vi "Planner_Creator.vi"(8 "error in (no error)":errorcluster) -> (0 "error out":errorcluster)   [LabVIEW 2017]
uses:
  <vilib>/Utility/file.llb/Read Delimited Spreadsheet (string).vi
  <vilib>/Utility/file.llb/Write Delimited Spreadsheet (string).vi
panel:
  out "Table":string[][](table)
  in  "BLOCK No":string(combo)
  in  "Delete Button":bool
  in  "Save Button":bool
  in  "Qty":u16=1 min=1 max=90 step=1
  in  "HOME":bool
  in  "UPDATE TABLE":bool
  in  "FG CAT No":string(combo)
  # "Plan Creater"
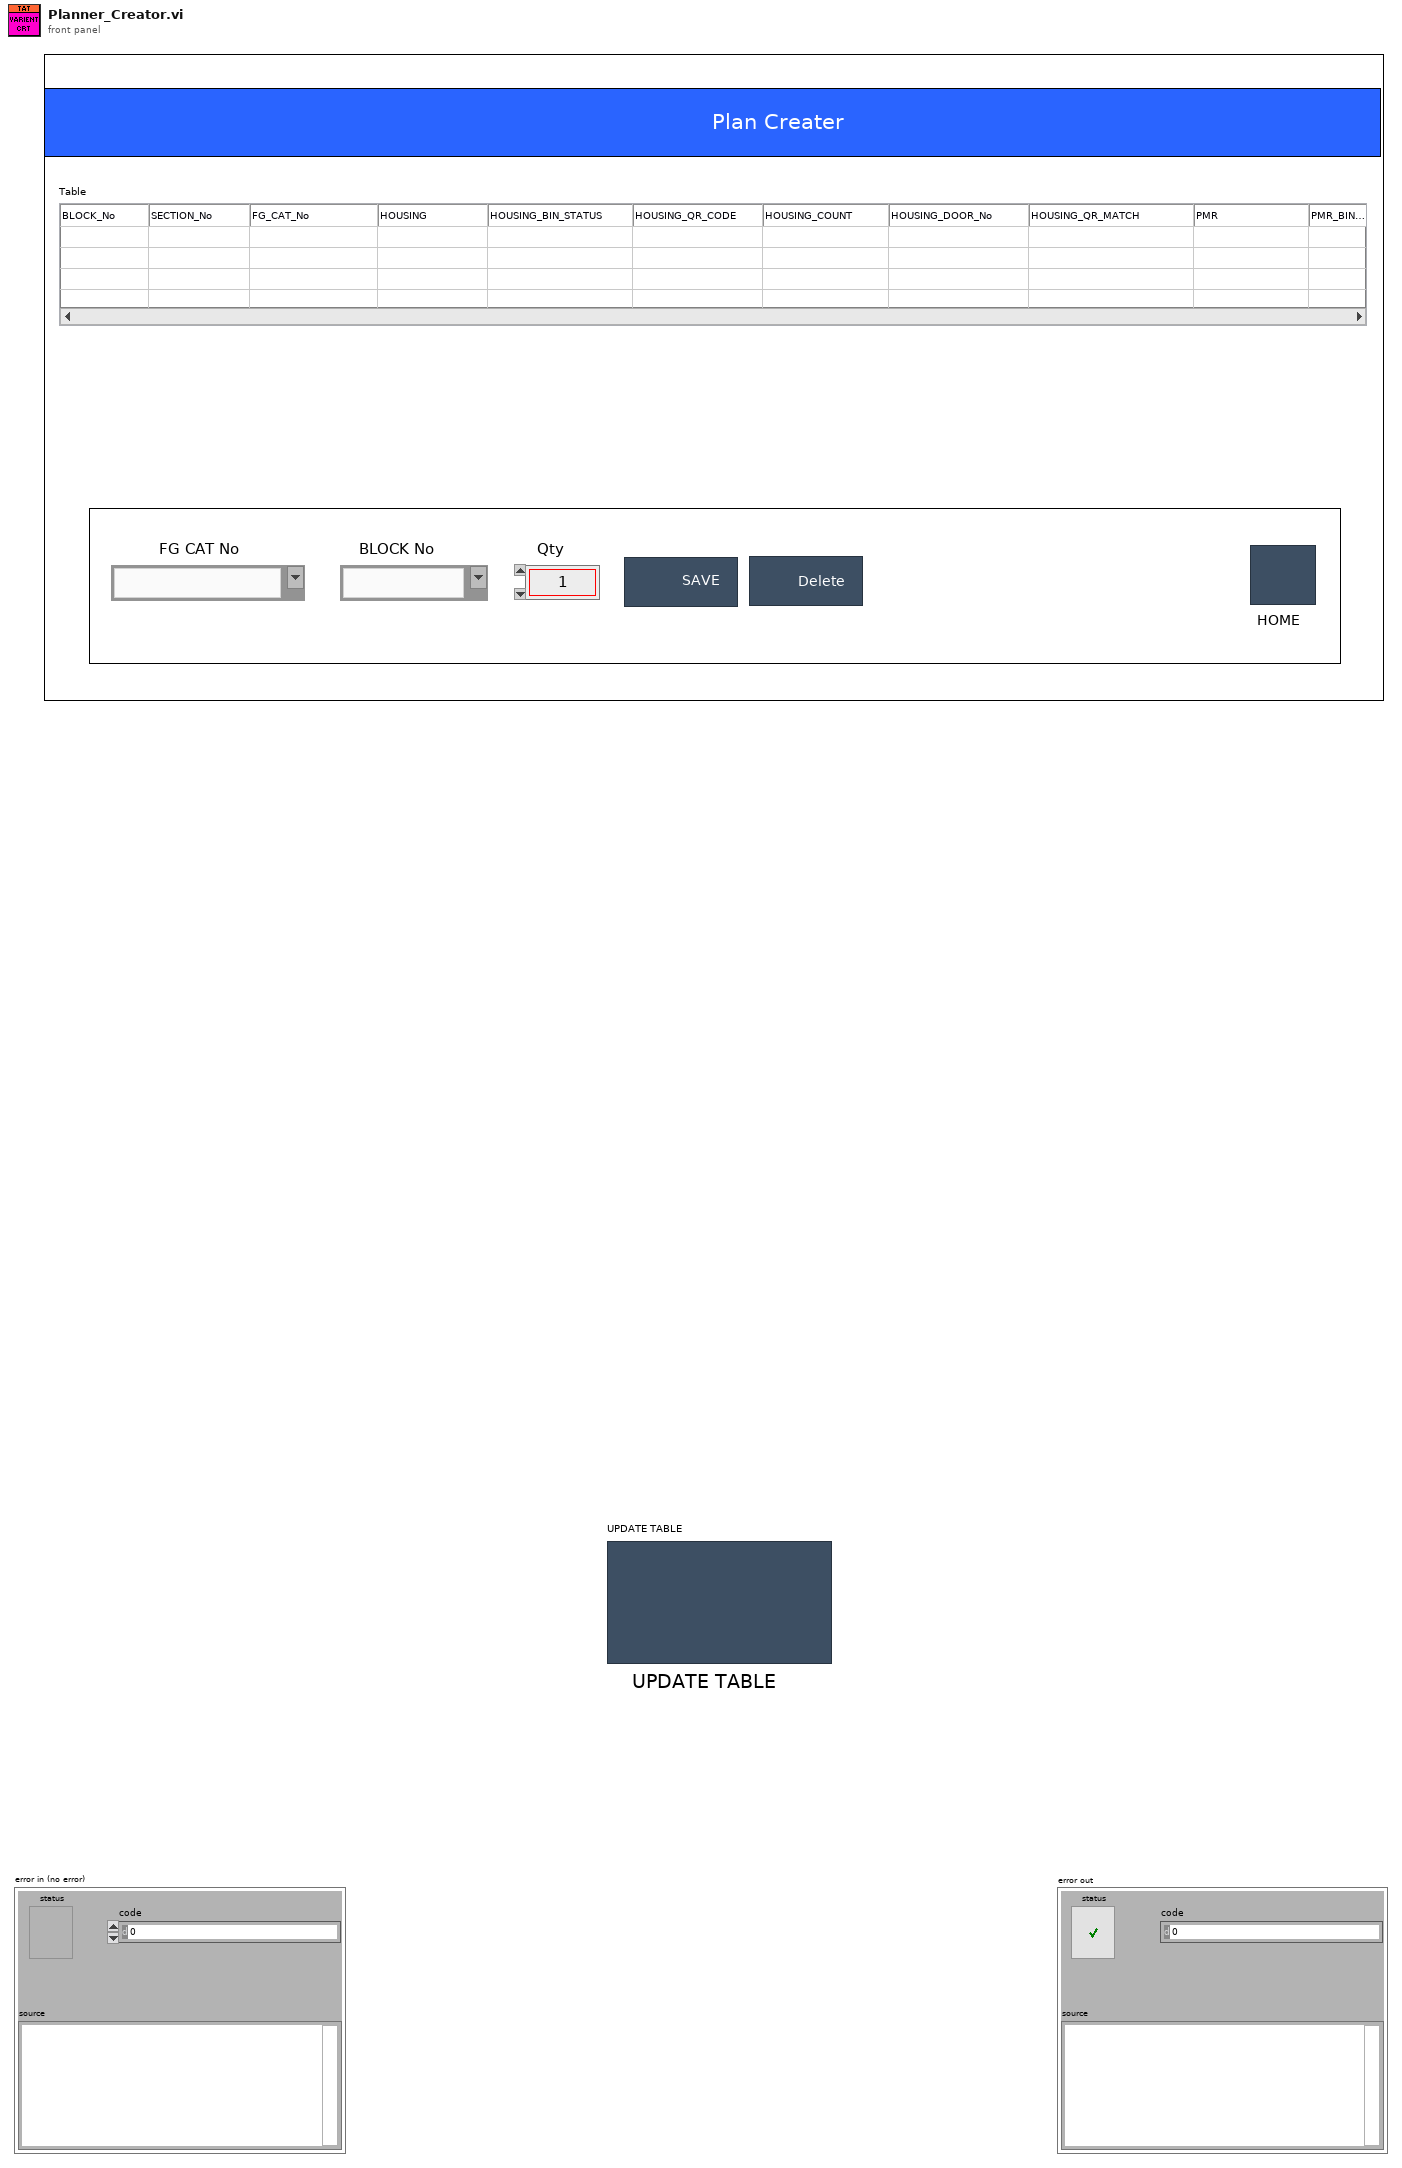
[diagram p1: front panel]
types:
  T1 = enum32{"invalid app kind", "Development System", "Run Time System", "Student Edition", "Embedded LabVIEW", "Evaluation", "Custom"}
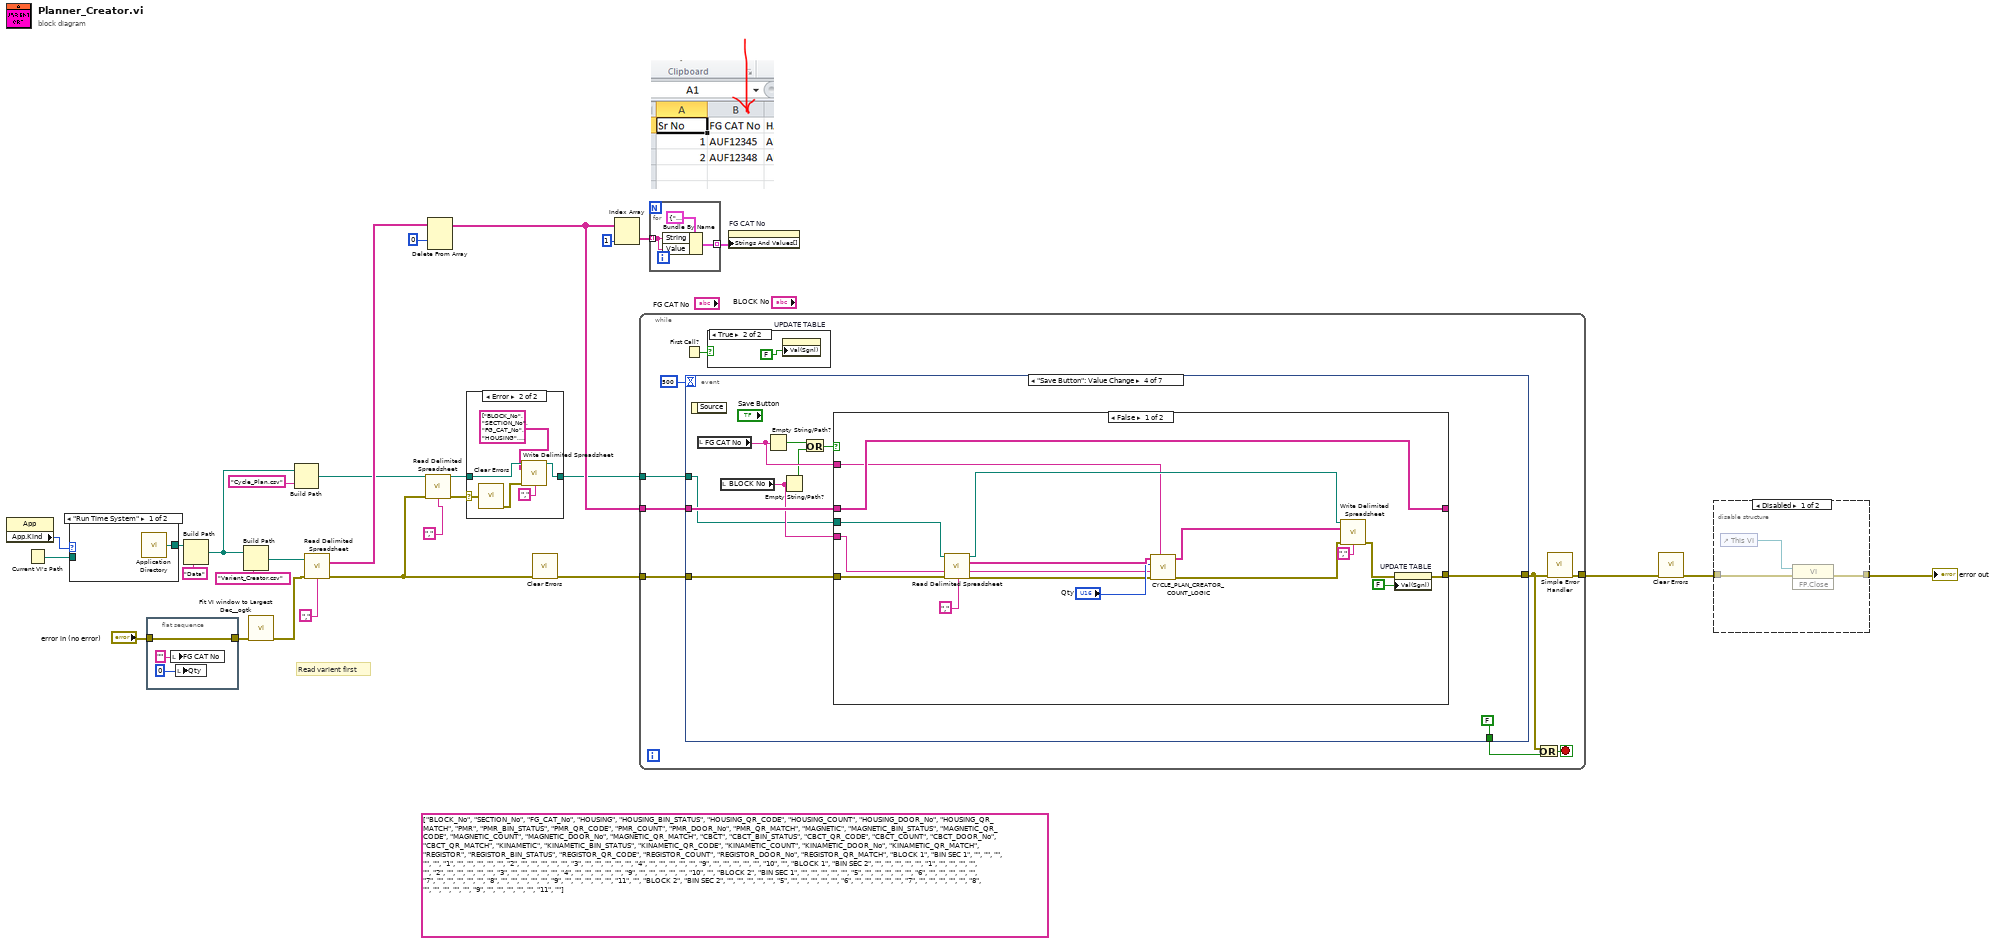
[diagram p0: block diagram]
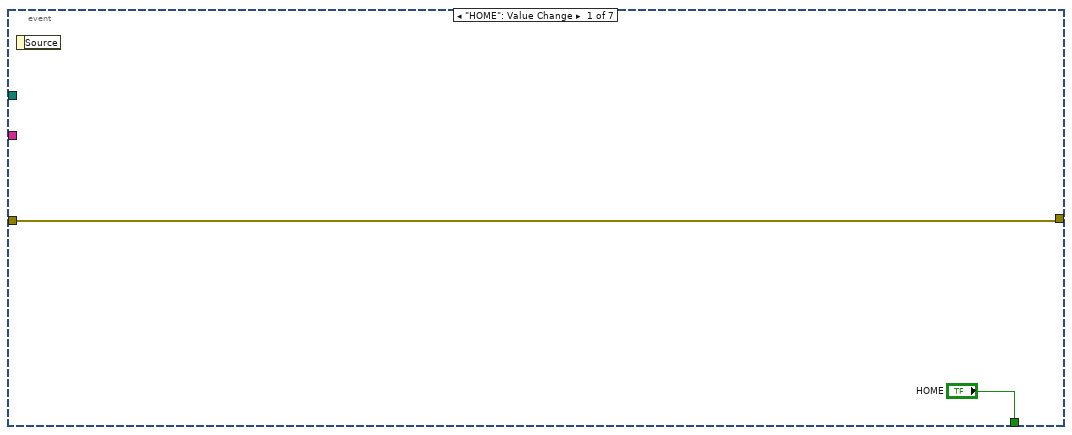
[diagram p4: hidden frame]
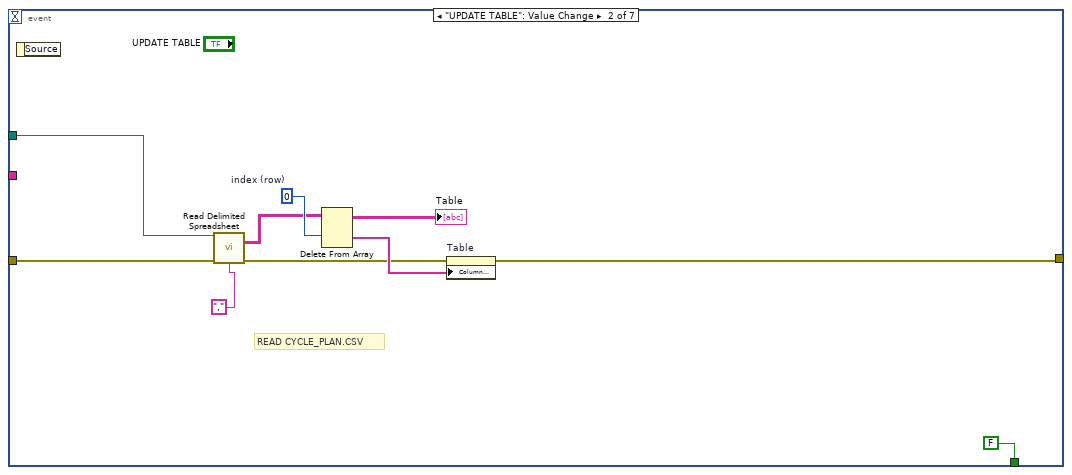
[diagram p5: hidden frame]
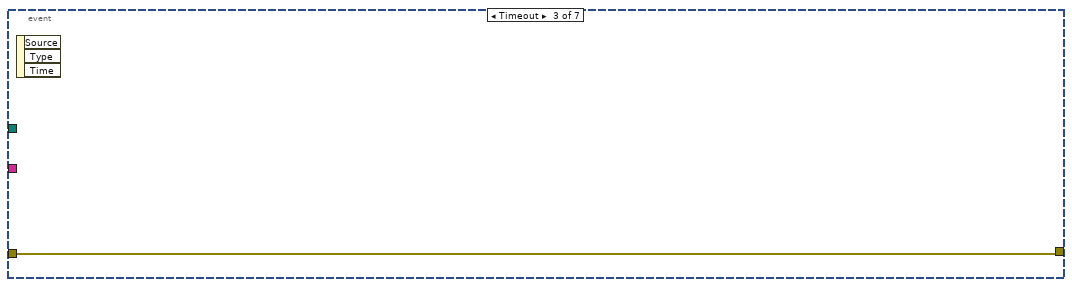
[diagram p6: hidden frame]
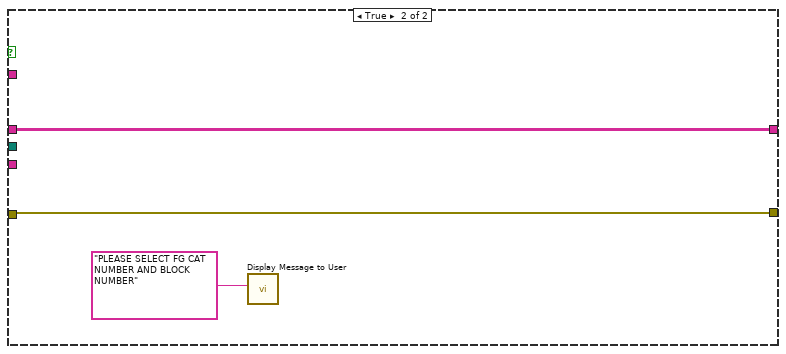
[diagram p7: hidden frame]
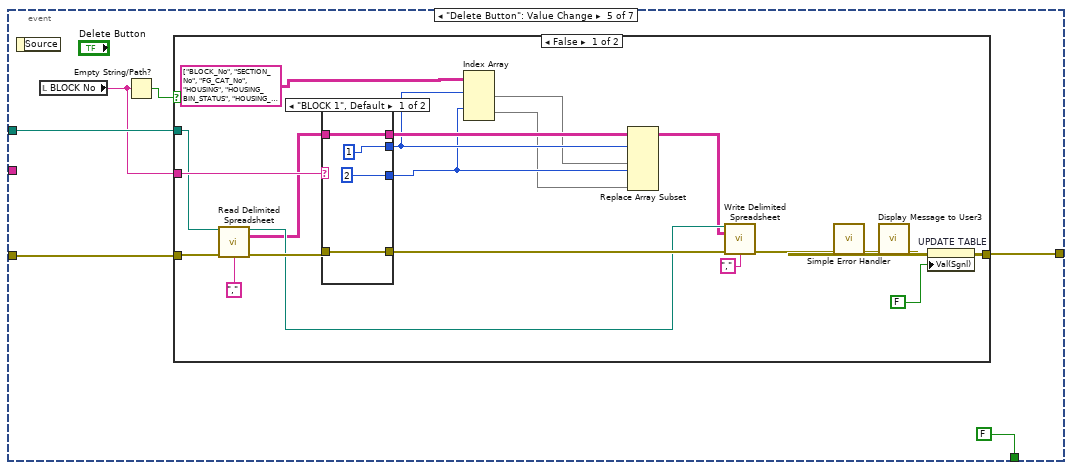
[diagram p8: hidden frame]
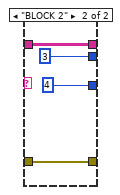
[diagram p9: hidden frame]
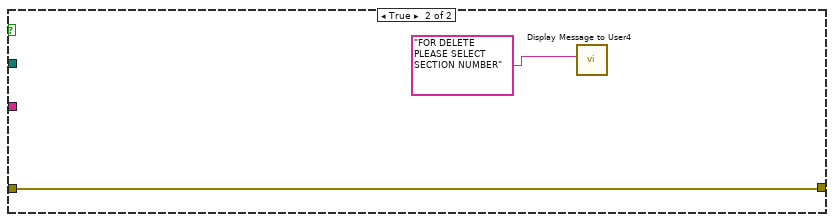
[diagram p10: hidden frame]
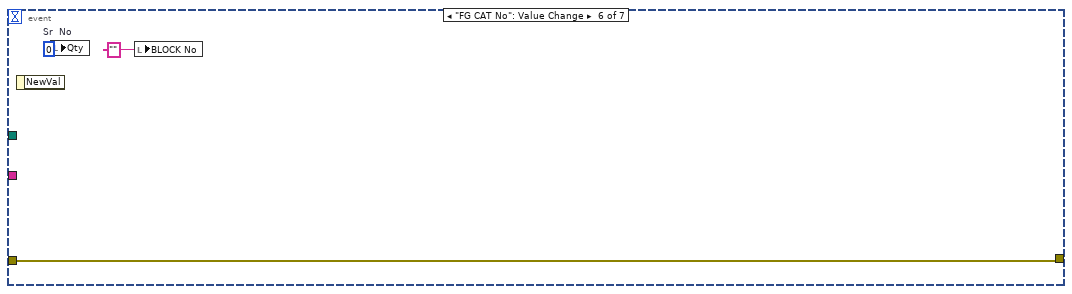
[diagram p11: hidden frame]
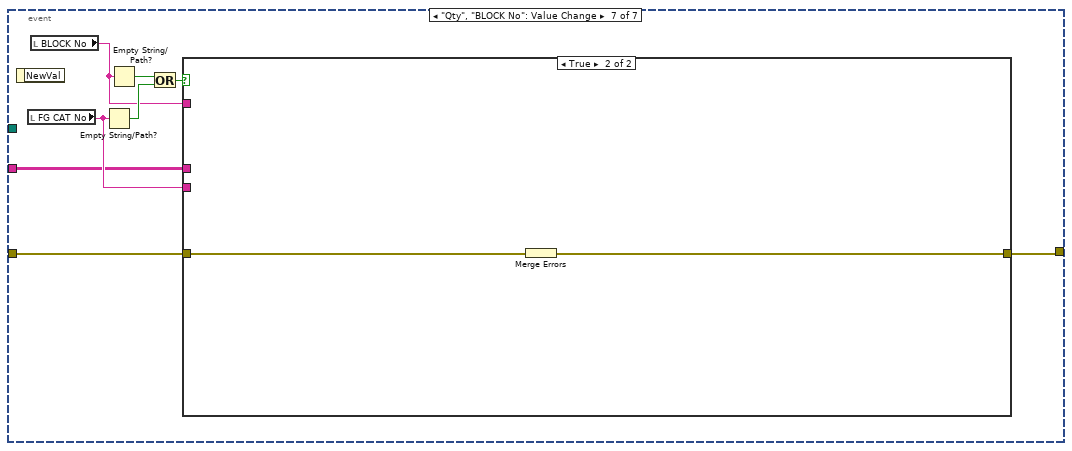
[diagram p12: hidden frame]
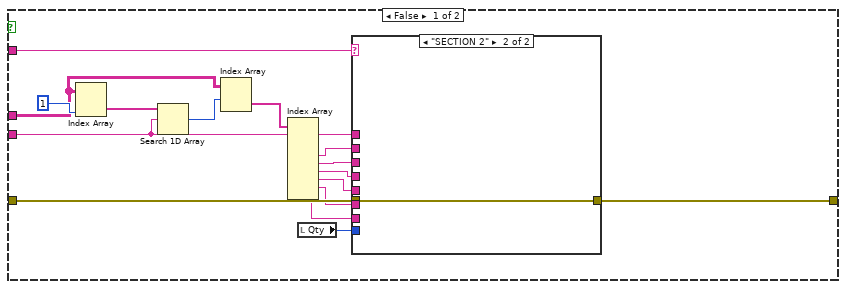
[diagram p13: hidden frame]
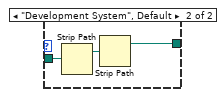
[diagram p16: hidden frame]
diagram:
  (unwired) string[][] [["BLOCK_No", "SECTION_No", "FG_CAT_No", "HOUSING", "HOUSING_BIN_STATUS", "HOUSING_QR_CODE", "HOUSING_COUNT", "HOUSING_DOOR_No", "HOUSING_QR_MATCH", "PMR", "PMR_BIN_STATUS", "PMR_QR_CODE", "PMR_COUNT", "PMR_DOOR_No", "PMR_QR_MATCH", "MAGNETIC", "MAGNETIC_BIN_STATUS", "MAGNETIC_QR_CODE", "MAGNETIC_COUNT", "MAGNETIC_DOOR_No", "MAGNETIC_QR_MATCH", "CBCT", "CBCT_BIN_STATUS", "CBCT_QR_CODE", "CBCT_COUNT", "CBCT_DOOR_No", "CBCT_QR_MATCH", "KINAMETIC", "KINAMETIC_BIN_STATUS", "KINAMETIC_QR_CODE", "KINAMETIC_COUNT", "KINAMETIC_DOOR_No", "KINAMETIC_QR_MATCH", "REGISTOR", "REGISTOR_BIN_STATUS", "REGISTOR_QR_CODE", "REGISTOR_COUNT", "REGISTOR_DOOR_No", "REGISTOR_QR_MATCH"], ["BLOCK 1", "BIN SEC 1", "", "", "", "", "", "1", "", "", "", "", "", "2", "", "", "", "", "", "3", "", "", "", "", "", "4", "", "", "", "", "", "9", "", "", "", "", "", "10", ""], ["BLOCK 1", "BIN SEC 2", "", "", "", "", "", "1", "", "", "", "", "", "2", "", "", "", "", "", "3", "", "", "", "", "", "4", "", "", "", "", "", "9", "", "", "", "", "", "10", ""], ["BLOCK 2", "BIN SEC 1", "", "", "", "", "", "5", "", "", "", "", "", "6", "", "", "", "", "", "7", "", "", "", "", "", "8", "", "", "", "", "", "9", "", "", "", "", "", "11", ""], ["BLOCK 2", "BIN SEC 2", "", "", "", "", "", "5", "", "", "", "", "", "6", "", "", "", "", "", "7", "", "", "", "", "", "8", "", "", "", "", "", "9", "", "", "", "", "", "11", ""]]
  # "Read varient first"
  n1 = property class="App"() -> ("App.Kind"=w22:T1)  [unwired: 2 in, 2 out]
  n2 = Current VI's Path() -> (path=w23:path)
  n3 = case shown="\"Run Time System\"" w22 {
    tunnel: w23 -> [_ w31]
    tunnel: [w29 w30] -> w19
    frame "Run Time System" {
      n4 = call <vilib>:"Application Directory.vi"() -> ("Application Directory"=w29:path)
    }
    frame "Development System", Default {
      n5 = Strip Path(path=w31) -> (stripped path=w32:path)  [unwired: 1 out]
      n6 = Strip Path(path=w32) -> (stripped path=w30:path)  [unwired: 1 out]
    }
  }
  n7 = flat-sequence {
    tunnel: [w35] -> w24
    tunnel: "error in (no error)" -> [w35]
    frame #0 {
      n8 = local write "FG CAT No"("" ("PART NUMBER")) -> ()
      n9 = local write "Qty"(u16 0 ("BATCH SIZE")) -> ()
    }
  }
  n10 = Build Path(base path=w19, name or relative path="Data") -> (appended path=w20:path)
  n11 = Build Path(base path=w20, name or relative path="Varient_Creator.csv") -> (appended path=w2:path)
  n12 = call <userlib>:"Fit VI window to Largest Dec__ogtk.vi"("error in (no error)"=w24) -> ("error out"=w18:errorcluster)  [unwired: 5 in, 1 out]
  n13 = Build Path(base path=w20, name or relative path="Cycle_Plan.csv") -> (appended path=w8:path)
  n14 = call-poly <vilib>:"Read Delimited Spreadsheet.vi"("file path (dialog if empty)"=w2, "error in (no error)"=w18, "delimiter (\\t)"=",") -> ("all rows"=w16:string[][], "error out"=w9:errorcluster)  [unwired: 7 in, 4 out]
  n15 = call-poly <vilib>:"Read Delimited Spreadsheet.vi"("file path (dialog if empty)"=w8, "error in (no error)"=w9, "delimiter (\\t)"=",") -> ("new file path (Not A Path if cancelled)"=w4:path, "error out"=w6:errorcluster)  [unwired: 7 in, 4 out]
  n16 = Delete From Array(array=w16, index (row)=0) -> (array with subset deleted=w11:string[][])  [unwired: 2 in, 1 out]
  n17 = case shown="Error" w6 {
    selector: w6 -> [_ w39]
    tunnel: [w36 w40] -> w5
    tunnel: w4 -> [w36 w41]
    frame No Error {
    }
    frame Error {
      n18 = call <vilib>:"Clear Errors.vi"("error in (no error)"=w39) -> ("error out"=w38:errorcluster)  [unwired: 5 in, 1 out]
      n19 = call-poly <vilib>:"Write Delimited Spreadsheet.vi"("file path (dialog if empty)"=w41, "2D data"=string[][] [["BLOCK_No", "SECTION_No", "FG_CAT_No", "HOUSING", "HOUSING_BIN_STATUS", "HOUSING_QR_CODE", "HOUSING_COUNT", "HOUSING_DOOR_No", "HOUSING_QR_MATCH", "PMR", "PMR_BIN_STATUS", "PMR_QR_CODE", "PMR_COUNT", "PMR_DOOR_No", "PMR_QR_MATCH", "MAGNETIC", "MAGNETIC_BIN_STATUS", "MAGNETIC_QR_CODE", "MAGNETIC_COUNT", "MAGNETIC_DOOR_No", "MAGNETIC_QR_MATCH", "CBCT", "CBCT_BIN_STATUS", "CBCT_QR_CODE", "CBCT_COUNT", "CBCT_DOOR_No", "CBCT_QR_MATCH", "KINAMETIC", "KINAMETIC_BIN_STATUS", "KINAMETIC_QR_CODE", "KINAMETIC_COUNT", "KINAMETIC_DOOR_No", "KINAMETIC_QR_MATCH", "REGISTOR", "REGISTOR_BIN_STATUS", "REGISTOR_QR_CODE", "REGISTOR_COUNT", "REGISTOR_DOOR_No", "REGISTOR_QR_MATCH"], ["BLOCK 1", "BIN SEC 1", "", "", "", "", "", "1", "", "", "", "", "", "2", "", "", "", "", "", "3", "", "", "", "", "", "4", "", "", "", "", "", "9", "", "", "", "", "", "10", ""], ["BLOCK 1", "BIN SEC 2", "", "", "", "", "", "1", "", "", "", "", "", "2", "", "", "", "", "", "3", "", "", "", "", "", "4", "", "", "", "", "", "9", "", "", "", "", "", "10", ""], ["BLOCK 2", "BIN SEC 1", "", "", "", "", "", "5", "", "", "", "", "", "6", "", "", "", "", "", "7", "", "", "", "", "", "8", "", "", "", "", "", "9", "", "", "", "", "", "11", ""], ["BLOCK 2", "BIN SEC 2", "", "", "", "", "", "5", "", "", "", "", "", "6", "", "", "", "", "", "7", "", "", "", "", "", "8", "", "", "", "", "", "9", "", "", "", "", "", "11", ""]], "error in (no error)"=w38, "delimiter (\\t)"=",") -> ("new file path (Not A Path if cancelled)"=w40:path)  [unwired: 10 in, 1 out]
    }
  }
  n20 = call <vilib>:"Clear Errors.vi"("error in (no error)"=w9) -> ("error out"=w10:errorcluster)  [unwired: 5 in, 1 out]
  n21 = Index Array(array=w11, index (col)=1) -> (element=w13:string[])  [unwired: 1 in]
  n22 = while {
    tunnel: [w46] -> w26
    tunnel: w10 -> [w48]
    tunnel: w11 -> [w44]
    tunnel: w5 -> [w43]
    stop <- w50 stop-if-true
    n23 = First Call?() -> (First Call?: T/F=w49:bool)
    n24 = event shown="[3] \"Save Button\": Value Change" {
      selector: _ -> [_ _ _ _ _ _ _]
      dyn-events: _ -> [_ _ _ _ _ _ _]
      timeout: 500 -> [_ _ _ _ _ _ _]
      tunnel: ["HOME" FALSE ("stop") _ FALSE ("stop") FALSE ("stop") _ _] -> w51
      tunnel: [w52 w54 w64 w72 w98 w132 w140] -> w47
      tunnel: w48 -> [w52 w61 w64 w71 w97 w132 w141]
      tunnel: w44 -> [_ _ _ w70 _ _ w134]
      tunnel: w43 -> [_ w60 _ w65 w96 _ _]
      event "HOME": Value Change {
        n25 = event-data() -> ()  [unwired: 1 in, 1 out]
      }
      event "UPDATE TABLE": Value Change {
        w59 = 0  # index (row)
        # "READ CYCLE_PLAN.CSV"
        n26 = event-data() -> ()  [unwired: 1 in, 1 out]
        n27 = call-poly <vilib>:"Read Delimited Spreadsheet.vi"("file path (dialog if empty)"=w60, "error in (no error)"=w61, "delimiter (\\t)"=",") -> ("all rows"=w57:string[][], "error out"=w55:errorcluster)  [unwired: 7 in, 4 out]
        n28 = Delete From Array(array=w57, index (row)=w59) -> (deleted portion=w58:string[], array with subset deleted=→"Table":string[][])  [unwired: 2 in]
        n29 = property on="Table" class="Tbl (strict)"(error in=w55, "Column Headers[]"=w58) -> (error out=w54:errorcluster)  [unwired: 1 in, 1 out]
      }
      event Timeout {
        n30 = event-data() -> ()  [unwired: 1 in, 3 out]
      }
      event "Save Button": Value Change {
        n31 = event-data() -> ()  [unwired: 1 in, 1 out]
        n32 = local read "FG CAT No"() -> (w73:string)
        n33 = local read "BLOCK No"() -> (w66:string)
        n34 = Empty String/Path?(string/path=w73) -> (empty?=w68:bool)
        n35 = Empty String/Path?(string/path=w66) -> (empty?=w69:bool)
        n36 = Or(x=w68, y=w69) -> (x .or. y?=w67:bool)
        n37 = case shown="False" w67 {
          tunnel: [w89 w92] -> w72
          tunnel: w73 -> [w79 _]
          tunnel: w71 -> [w84 w92]
          tunnel: w70 -> [w88 w91]
          tunnel: [w88 w91] -> _
          tunnel: w66 -> [w77 _]
          tunnel: w65 -> [w83 _]
          frame False {
            n38 = call-poly <vilib>:"Read Delimited Spreadsheet.vi"("file path (dialog if empty)"=w83, "error in (no error)"=w84, "delimiter (\\t)"=",") -> ("new file path (Not A Path if cancelled)"=w82:path, "all rows"=w81:string[][], "error out"=w78:errorcluster)  [unwired: 7 in, 3 out]
            n39 = call "CYCLE_PLAN_CREATOR_COUNT_LOGIC.vi"("FG CAT No"=w79, "error in (no error)"=w78, "BLOCK NO"=w77, "Qty"="Qty", "all rows IN"=w81) -> ("error out"=w75:errorcluster, "all rows OUT"=w76:string[][])  [unwired: 5 in]
            n40 = call-poly <vilib>:"Write Delimited Spreadsheet.vi"("file path (dialog if empty)"=w82, "2D data"=w76, "error in (no error)"=w75, "delimiter (\\t)"=",") -> ("error out"=w87:errorcluster)  [unwired: 10 in, 1 out]
            n41 = property on="UPDATE TABLE" class="Bool (strict)"(error in=w87, "Val(Sgnl)"=FALSE) -> (error out=w89:errorcluster)  [unwired: 1 in, 1 out]
          }
          frame True {
            n42 = call "Display Message to User"("Message"="PLEASE SELECT FG CAT NUMBER AND BLOCK NUMBER") -> ()  [unwired: 9 in, 2 out]
          }
        }
      }
      event "Delete Button": Value Change {
        n43 = event-data() -> ()  [unwired: 1 in, 1 out]
        n44 = local read "BLOCK No"() -> (w95:string)
        n45 = Empty String/Path?(string/path=w95) -> (empty?=w94:bool)
        n46 = case shown="False" w94 {
          tunnel: [w119 w129] -> w98
          tunnel: w97 -> [w115 w129]
          tunnel: w95 -> [w116 _]
          tunnel: w96 -> [w112 _]
          frame False {
            n47 = call-poly <vilib>:"Read Delimited Spreadsheet.vi"("file path (dialog if empty)"=w112, "error in (no error)"=w115, "delimiter (\\t)"=",") -> ("new file path (Not A Path if cancelled)"=w108:path, "all rows"=w106:string[][], "error out"=w114:errorcluster)  [unwired: 7 in, 3 out]
            n48 = case shown="\"BLOCK 1\", Default" w116 {
              tunnel: w114 -> [w124 w128]
              tunnel: [w124 w128] -> w110
              tunnel: [w123 w127] -> w107
              tunnel: w106 -> [w123 w127]
              tunnel: [1 ("disabled index (col)") 3 ("disabled index (col)")] -> w104
              tunnel: [2 ("disabled index (col)") 4 ("disabled index (col)")] -> w103
              frame "BLOCK 1", Default {
              }
              frame "BLOCK 2" {
              }
            }
            n49 = Index Array(array=string[][] [["BLOCK_No", "SECTION_No", "FG_CAT_No", "HOUSING", "HOUSING_BIN_STATUS", "HOUSING_QR_CODE", "HOUSING_COUNT", "HOUSING_DOOR_No", "HOUSING_QR_MATCH", "PMR", "PMR_BIN_STATUS", "PMR_QR_CODE", "PMR_COUNT", "PMR_DOOR_No", "PMR_QR_MATCH", "MAGNETIC", "MAGNETIC_BIN_STATUS", "MAGNETIC_QR_CODE", "MAGNETIC_COUNT", "MAGNETIC_DOOR_No", "MAGNETIC_QR_MATCH", "CBCT", "CBCT_BIN_STATUS", "CBCT_QR_CODE", "CBCT_COUNT", "CBCT_DOOR_No", "CBCT_QR_MATCH", "KINAMETIC", "KINAMETIC_BIN_STATUS", "KINAMETIC_QR_CODE", "KINAMETIC_COUNT", "KINAMETIC_DOOR_No", "KINAMETIC_QR_MATCH", "REGISTOR", "REGISTOR_BIN_STATUS", "REGISTOR_QR_CODE", "REGISTOR_COUNT", "REGISTOR_DOOR_No", "REGISTOR_QR_MATCH"], ["BLOCK 1", "BIN SEC 1", "", "", "", "", "", "1", "", "", "", "", "", "2", "", "", "", "", "", "3", "", "", "", "", "", "4", "", "", "", "", "", "9", "", "", "", "", "", "10", ""], ["BLOCK 1", "BIN SEC 2", "", "", "", "", "", "1", "", "", "", "", "", "2", "", "", "", "", "", "3", "", "", "", "", "", "4", "", "", "", "", "", "9", "", "", "", "", "", "10", ""], ["BLOCK 2", "BIN SEC 1", "", "", "", "", "", "5", "", "", "", "", "", "6", "", "", "", "", "", "7", "", "", "", "", "", "8", "", "", "", "", "", "9", "", "", "", "", "", "11", ""], ["BLOCK 2", "BIN SEC 2", "", "", "", "", "", "5", "", "", "", "", "", "6", "", "", "", "", "", "7", "", "", "", "", "", "8", "", "", "", "", "", "9", "", "", "", "", "", "11", ""]], index (row) #1=w104, index (row) #2=w103) -> (element #1=w102:string[], element #2=w101:string[])  [unwired: 2 in]
            n50 = Replace Array Subset(array=w107, new element #1=w102, index (row) #1=w104, new element #2=w101, index (row) #2=w103) -> (w105:string[][])  [unwired: 2 in]
            n51 = call-poly <vilib>:"Write Delimited Spreadsheet.vi"("file path (dialog if empty)"=w108, "2D data"=w105, "error in (no error)"=w110, "delimiter (\\t)"=",") -> ("error out"=w109:errorcluster)  [unwired: 10 in, 1 out]
            n52 = call <vilib>:"Simple Error Handler.vi"("error in (no error)"=w109) -> ("error out"=w118:errorcluster)  [unwired: 4 in, 4 out]
            n53 = call "Display Message to User3"("error in (no error)"=w118) -> ("error out"=w117:errorcluster)  [unwired: 9 in, 1 out]
            n54 = property on="UPDATE TABLE" class="Bool (strict)"(error in=w117, "Val(Sgnl)"=FALSE) -> (error out=w119:errorcluster)  [unwired: 1 in, 1 out]
          }
          frame True {
            n55 = call "Display Message to User4"("Message"="FOR DELETE PLEASE SELECT SECTION NUMBER") -> ()  [unwired: 9 in, 2 out]
          }
        }
      }
      event "FG CAT No": Value Change {
        w133 = u16 0  # Sr  No
        n56 = event-data() -> ()  [unwired: 1 in, 1 out]
        n57 = local write "Qty"(w133) -> ()
        n58 = local write "BLOCK No"("") -> ()
      }
      event "Qty", "BLOCK No": Value Change {
        n59 = event-data() -> ()  [unwired: 1 in, 1 out]
        n60 = local read "FG CAT No"() -> (w136:string)
        n61 = local read "BLOCK No"() -> (w135:string)
        n62 = Empty String/Path?(string/path=w136) -> (empty?=w138:bool)
        n63 = Empty String/Path?(string/path=w135) -> (empty?=w139:bool)
        n64 = Or(x=w139, y=w138) -> (x .or. y?=w137:bool)
        n65 = case shown="True" w137 {
          tunnel: w141 -> [w157 w161]
          tunnel: [w156 w160] -> w140
          tunnel: w135 -> [w155 _]
          tunnel: w136 -> [w152 _]
          tunnel: w134 -> [w149 _]
          frame False {
            n66 = Index Array(array=w149, index (col)=1) -> (element=w151:string[])  [unwired: 1 in]
            n67 = Search 1D Array(1D array=w151, element=w152) -> (index of element=w150:i32)  [unwired: 1 in]
            n68 = Index Array(array=w149, index (row)=w150) -> (element=w148:string[])  [unwired: 1 in]
            n69 = Index Array(array=w148) -> (element #3=w147:string, element #4=w146:string, element #5=w145:string, element #6=w144:string, element #7=w143:string, element #8=w142:string)  [unwired: 8 in, 2 out]
            n70 = local read "Qty"() -> (w154:u16)
            n71 = case shown="\"SECTION 2\"" w155 {
              tunnel: w157 -> [w158 w159]
              tunnel: [w158 w159] -> w156
              tunnel: w152 -> [_ _]
              tunnel: w154 -> [_ _]
              tunnel: w147 -> [_ _]
              tunnel: w146 -> [_ _]
              tunnel: w145 -> [_ _]
              tunnel: w144 -> [_ _]
              tunnel: w143 -> [_ _]
              tunnel: w142 -> [_ _]
              frame "SECTION 1", Default {
              }
              frame "SECTION 2" {
              }
            }
          }
          frame True {
            n72 = Merge Errors(w161) -> (w160:errorcluster)
          }
        }
      }
    }
    n73 = case shown="True" w49 {
      frame False {
      }
      frame True {
        n74 = property on="UPDATE TABLE" class="Bool (strict)"("Val(Sgnl)"=FALSE) -> ()  [unwired: 2 in, 2 out]
      }
    }
    n75 = Or(x=w47, y=w51) -> (x .or. y?=w50:bool)
    n76 = call <vilib>:"Simple Error Handler.vi"("error in (no error)"=w47) -> ("error out"=w46:errorcluster)  [unwired: 4 in, 4 out]
  }
  n77 = for {
    tunnel: w13 -> [w164] mode=indexing
    tunnel: [w163] -> w12 mode=indexing
    n78 = Bundle By Name(cluster=cluster{"String":string, "Value":string} {"String"="", "Value"=""}, "String"=w164, "Value"=w164) -> (w163:cluster{"String":string, "Value":string})
  }
  n79 = property on="FG CAT No" class="CmbBox"("Strings And Values[]"=w12) -> ()  [unwired: 2 in, 2 out]
  n80 = call <vilib>:"Clear Errors.vi"("error in (no error)"=w26) -> ("error out"=w28:errorcluster)  [unwired: 5 in, 1 out]
  n81 = disable-structure shown="Disabled" {
    disable-tunnel: w28 -> [w168 w169]
    disable-tunnel: [w167 w169] -> w27
    frame Disabled {
      n82 = control-ref of="This VI"() -> (w166:refnum<vi>)
      n83 = invoke class="VI" method="FP.Close"(reference=w166, error in=w168) -> (error out=w167:errorcluster)  [unwired: 1 in, 2 out]
    }
    frame Enabled {
    }
  }
  "error out" <- w27
